vi "Ultrasonic Read Fixed.vi"(8 "Error In":errorcluster, 9 "DO Channel":u8, 10 "DI Channel":u8, 11 "LINX Resource":T1) -> (0 "Error Out":errorcluster, 1 "Centimeters":dbl, 2 "Inches":dbl, 3 "LINX Resource":T1)   [LabVIEW 2019]
uses:
  <vilib>/MakerHub/LINX/Private/Type Defs/LINX Ref.ctl
  <vilib>/MakerHub/LINX/Private/Type Defs/Platform.ctl
  <vilib>/MakerHub/LINX/Private/Type Defs/Interface.ctl
  <vilib>/MakerHub/LINX/Private/Device/Type Defs/LINX Device Config.ctl
  <vilib>/MakerHub/LINX/Private/Device/Type Defs/TCP Config.ctl
  <vilib>/MakerHub/LINX/Private/Device/Type Defs/Channels.ctl
  <vilib>/MakerHub/LINX/Private/Device/Type Defs/Stimulus Pulse.ctl
  <vilib>/MakerHub/LINX/Private/Device/Type Defs/Pulse Polarity.ctl
  <vilib>/MakerHub/LINX/LMH-LINX.lvlib
  <vilib>/MakerHub/LINX/Private/Device/Device.lvlib
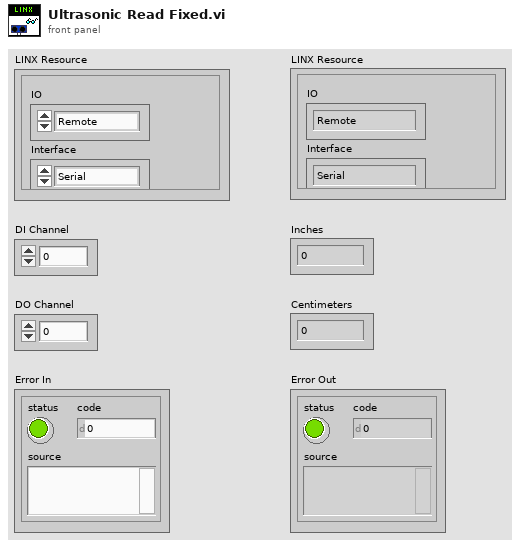
[diagram p1: front panel]
types:
  T1 = typedef "LMH-LINX.lvlib/LINX Ref.ctl" = cluster{"IO":T2, "Interface":T3, "LINX Device Config":T4}
  T2 = typedef "LMH-LINX.lvlib/Platform.ctl" = enum16{"Remote", "Local"}
  T3 = typedef "LMH-LINX.lvlib/Interface.ctl" = enum16{"Serial", "TCP"}
  T4 = typedef "LMH-LINX.lvlib/Device.lvlib/LINX Device Config.ctl" = cluster{"Interface":T3, "COM Port":refnum<visa-resource-name>, "TCP Configuration":T5, "Device Family":u8, "Device ID":u8, "Device Name":string, "TCP Ref":refnum<k5>, "Channels":T6}
  T5 = typedef "LMH-LINX.lvlib/Device.lvlib/TCP Config.ctl" = cluster{"IP Address":string, "Port":u16}
  T6 = typedef "LMH-LINX.lvlib/Channels.ctl" = cluster{"DI":u8[], "DO":u8[], "AI":u8[], "AO":u8[], "PWM":u8[], "QE":u8[], "UART":u8[], "I2C 2":u8[], "SPI":u8[], "CAN":u8[], "Servo":u8[], "AI Ref (V)":dbl, "AI Resolution (Bits)":u8, "AO Ref (V)":dbl, "AO Resolution (Bits)":u8}
  T7 = typedef "LMH-LINX.lvlib/Device.lvlib/Pulse Polarity.ctl" = enum8{"Active Low", "Active High"}
  T8 = typedef "LMH-LINX.lvlib/Device.lvlib/Stimulus Pulse.ctl" = enum16{"None", "Active Low", "Active High"}
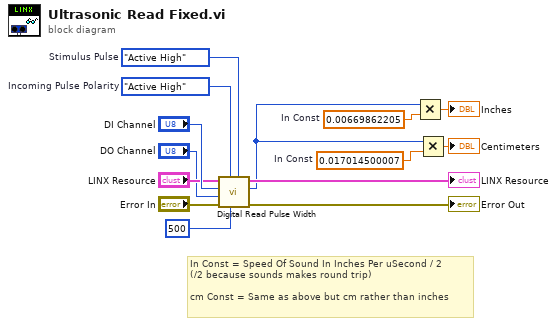
[diagram p0: block diagram]
diagram:
  w1 = Pulse_Polarity."Active High"  # Incoming Pulse Polarity
  w2 = Stimulus_Pulse."Active High"  # Stimulus Pulse
  w4 = 0.017014500007  # In Const
  w8 = 0.00669862205  # In Const
  # "In Const = Speed Of Sound In Inches Per uSecond / 2\n(/2 because sounds makes round trip)\n\ncm Const = Same as above but cm rather than inches"
  n1 = call <vilib>:"Digital Read Pulse Width.vi"("Stimulus Pulse (Active High)"=w2, "Timeout  (250 mS)"=u32 500, "Incoming Pulse Polarity (Active High)"=w1, "Error In"="Error In", "DO Channel"="DO Channel", "DI Channel"="DI Channel", "LINX Resource"="LINX Resource") -> ("Error Out"=→"Error Out":errorcluster, "Pulse Width (uS)"=w5:u32, "LINX Resource"=→"LINX Resource":T1)  [unwired: 2 in]
  n2 = Multiply(x=w5, y=w8) -> (x*y=→"Inches":dbl)
  n3 = Multiply(x=w5, y=w4) -> (x*y=→"Centimeters":dbl)
